vi "SavLogGen.vi"(7 "CheminSauv":path=path "C:/Données/Run003" caption="Fichier de Sauvegarde", 8 "error in":errorcluster, 10 "DonnéesY":dbl[](array[numeric]), 11 "NouvTemps":dbl) -> (0 "error out":errorcluster, 2 "DonnéesY out":dbl[](array[numeric]), 3 "NouvTemps Out":dbl)   [LabVIEW 2019]
doc: "Ce Vi sauvegarde les données sous forme de collonnes dans le fichier texte de sauvegarde"
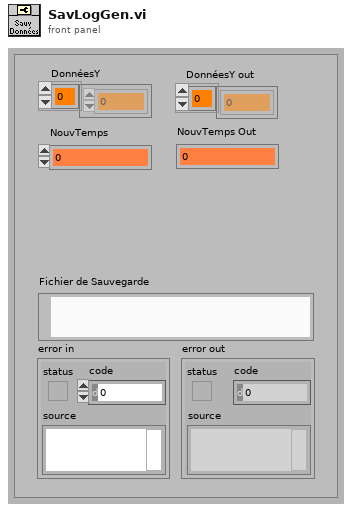
[diagram p1: front panel]
types:
  T1 = enum16{"open", "open or create", "create or replace", "create", "open (read only)"}
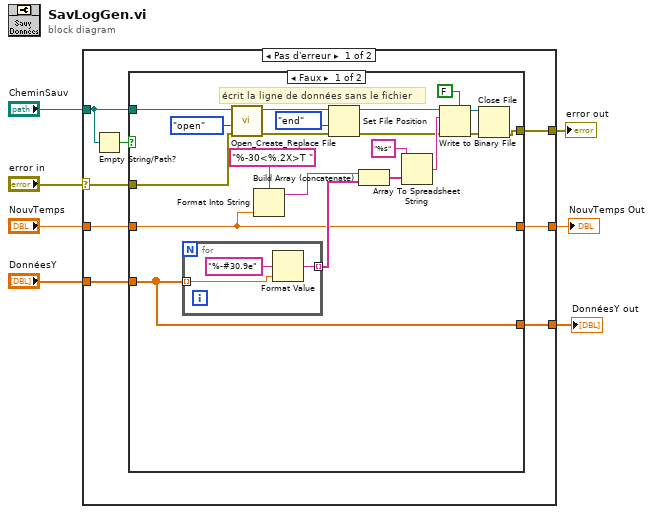
[diagram p0: block diagram]
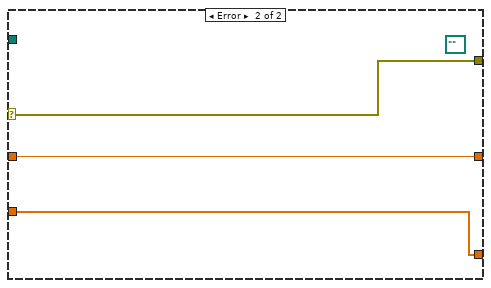
[diagram p3: hidden frame]
diagram:
  n1 = case shown="Pas d'erreur" "error in" {
    selector: "error in" -> [w14 w44]
    tunnel: [w15 w44] -> w7
    tunnel: "CheminSauv" -> [w10 _]
    tunnel: "DonnéesY" -> [w12 w43]
    tunnel: "NouvTemps" -> [w13 w42]
    tunnel: [w8 w42] -> w2
    tunnel: [w9 w43] -> w1
    frame No Error {
      n2 = Empty String/Path?(string/path=w10) -> (empty?=w11:bool)
      n3 = case shown="Faux" w11 {
        tunnel: [w30 w41] -> w15
        tunnel: w14 -> [w29 w41]
        tunnel: w10 -> [w28 _]
        tunnel: w13 -> [w16 w40]
        tunnel: w12 -> [w22 w39]
        tunnel: [w22 w39] -> w9
        tunnel: [w16 w40] -> w8
        frame False {
          # "écrit la ligne de données sans le fichier"
          n4 = for {
            tunnel: w22 -> [w37] mode=indexing
            tunnel: [w36] -> w26 mode=indexing
            n5 = Format Value(format string="%-#30.9e", value (0)=w37) -> (output string=w36:string)  [unwired: 1 in]
          }
          n6 = call <vilib>:"Open_Create_Replace File.vi"("error in (no error)"=w29, "function (open:0)"=T1."open", "file path"=w28) -> ("error out"=w35:errorcluster, "refnum"=w31:refnum<file>)  [unwired: 5 in, 2 out]
          n7 = Format Into String(format string="%-30<%.2X>T " ("chaîne de format"), w16) -> (resulting string=w17:string)  [unwired: 2 in, 1 out]
          n8 = Set File Position(refnum=w31, from (0:start)=enum16{"start", "end", "current"}."end" ("pos mode (0:2)"), error in=w35) -> (refnum out=w21:refnum<file>, error out=w20:errorcluster)  [unwired: 1 in]
          n9 = Build Array (concatenate)(w17, w26) -> (w25:string[])
          n10 = Array To Spreadsheet String(array=w25, 3:"%s" ("format string")) -> (spreadsheet string=w23:string)  [unwired: 1 in]
          n11 = Write to Binary File(file (use dialog)=w21, data=w23, error in=w20, 5:FALSE ("ajouter une taille de tableau ou de chaîne ? (V)")) -> (refnum out=w32:refnum<file>, error out=w34:errorcluster)  [unwired: 2 in, 1 out]
          n12 = Close File(refnum=w32, error in=w34) -> (error out=w30:errorcluster)  [unwired: 1 out]
        }
        frame True {
          # "path vide: on ne sauvegarde pas"
        }
      }
    }
    frame Error {
      (unwired) path "" ("path")
    }
  }
  "error out" <- w7
  "NouvTemps Out" <- w2
  "DonnéesY out" <- w1
